vi "niRFSG Configure RF.vi"(0 "instrument handle":refnum<k15>, 5 "frequency (Hz)":dbl=100000000.0 format="%.2p", 7 "power level (dBm)":dbl=-90.0 format="%.2f", 11 "error in":errorcluster {"code" format="%.0x"}) -> (4 "instrument handle out":refnum<k15>, 15 "error out":errorcluster {"code" format="%.0x"})   [LabVIEW 2014]
doc: "Configures the frequency and power level of the RF output signal. The NI 5670/5671/5672 device must be in the Configuration state before you call this VI. The NI 5644R/5645R/5646R/5650/5651/5652/5654/5654 with NI 5696/5673/5673E/5840 device can be in the Configuration state or Generation state when you call this VI.\n\n<B>Supported Devices</B>: NI 5644R/5645R/5646R, NI 5650/5651/5652/5654/5654 with NI 5696, NI 5670/5671/5672/5673/5673E, NI 5840"
uses:
  niRFSG.dll
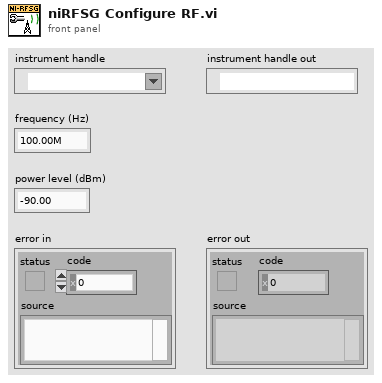
[diagram p1: front panel]
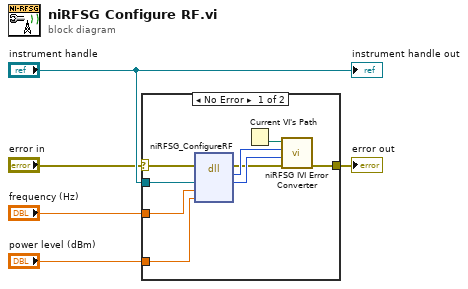
[diagram p0: block diagram]
diagram:
  n1 = case shown="No Error" "error in" {
    selector: "error in" -> [w9 w15]
    tunnel: "instrument handle" -> [w14 _]
    tunnel: [w13 w15] -> w3
    tunnel: "frequency (Hz)" -> [w7 _]
    tunnel: "power level (dBm)" -> [w6 _]
    frame No Error {
      n2 = dll-call lib="niRFSG**.*" fn="niRFSG_ConfigureRF"(error in=w9, "instrument handle"=w14, "Frequency"=w7, "Power Level"=w6) -> (error out=w8:errorcluster, "status"=w11:i32, "instrument handle"=w10:u32)  [unwired: 4 in, 1 out]
      n3 = Current VI's Path() -> (path=w12:path)
      n4 = call "niRFSG IVI Error Converter.vi"("error in"=w8, "instrument handle"=w10, "IVI error code"=w11, "path to VI"=w12) -> ("error out"=w13:errorcluster)  [unwired: 7 in]
    }
    frame Error {
    }
  }
  "error out" <- w3
  "instrument handle out" <- "instrument handle"
